vi "GetDataTDCV775_D32.vi"(8 "error in (no error)":errorcluster, 10 "handle in":i32, 11 "VME Base Address":u32) -> (0 "error out":errorcluster, 1 "Time Elapsed":u16, 2 "handle out":i32, 3 "Array":u32[](array[numeric]))   [LabVIEW 2014]
uses:
  Program Files (x86)/CAEN/Comm/labview/CAENComm.lvlib
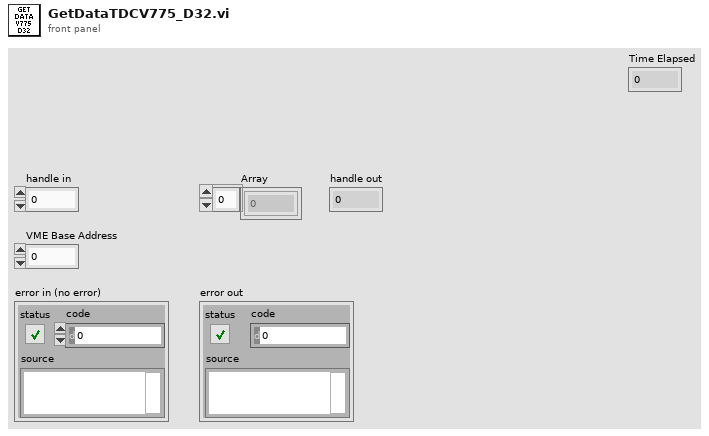
[diagram p1: front panel]
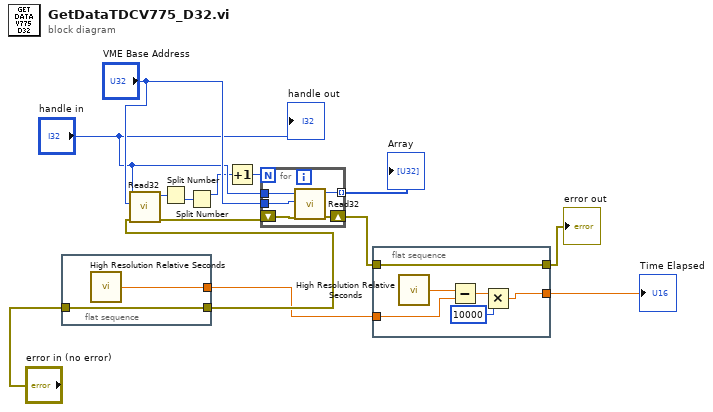
[diagram p0: block diagram]
diagram:
  n1 = flat-sequence {
    tunnel: "error in (no error)" -> [w16]
    tunnel: [w16] -> w5
    tunnel: [w15] -> w2
    frame #0 {
      n2 = call <vilib>:"High Resolution Relative Seconds.vi"() -> ("relative seconds"=w15:dbl)
    }
  }
  n3 = call "Read32.vi"("error in (no error)"=w5, "Address"="VME Base Address", "handle"="handle in") -> ("error out"=w8:errorcluster, "Data"=w9:u32)  [unwired: 7 in]
  n4 = Split Number(x=w9) -> (lo(x)=w10:u16)  [unwired: 1 out]
  n5 = Split Number(x=w10) -> (hi(x)=w12:u8)  [unwired: 1 out]
  n6 = Increment(x=w12) -> (x+1=w11:u8)
  n7 = for {
    N: w11 -> [_]
    shift-right: [w20] -> w3
    shift-left: w8 -> [w21]
    tunnel: "handle in" -> [w19]
    tunnel: "VME Base Address" -> [w18]
    tunnel: [w17] -> w7 mode=indexing
    n8 = call "Read32.vi"("error in (no error)"=w21, "Address"=w18, "handle"=w19) -> ("error out"=w20:errorcluster, "Data"=w17:u32)  [unwired: 7 in]
  }
  "Array" <- w7
  n9 = flat-sequence {
    tunnel: [w27] -> w4
    tunnel: w3 -> [w27]
    tunnel: w2 -> [w25]
    tunnel: [w22] -> w1
    frame #0 {
      n10 = call <vilib>:"High Resolution Relative Seconds.vi"() -> ("relative seconds"=w26:dbl)
      n11 = Subtract(x=w26, y=w25) -> (x-y=w24:dbl)
      n12 = Multiply(x=w24, y=u16 10000) -> (x*y=w22:dbl)
    }
  }
  "error out" <- w4
  "handle out" <- "handle in"
  "Time Elapsed" <- w1
